vi "raise Height state.vi"(8 "Write Height":dbl, 9 "Write":bool, 11 "Enum":enum16{"read", "write"}(ring)) -> (0 "read Height":dbl, 1 "read":bool)   [LabVIEW 2019]
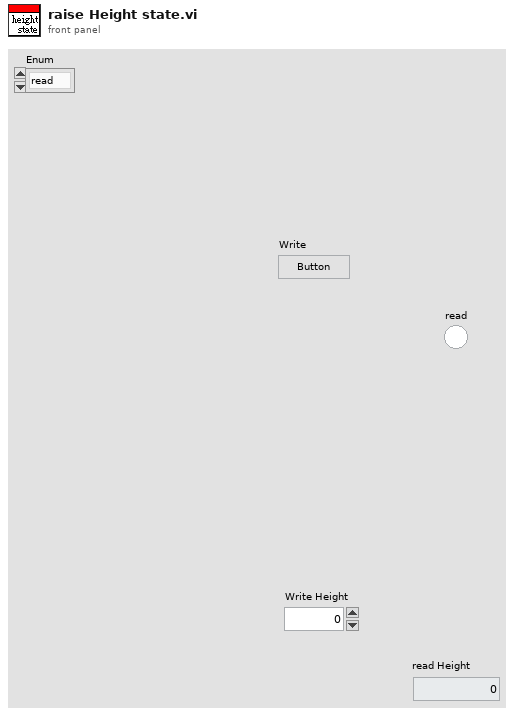
[diagram p1: front panel]
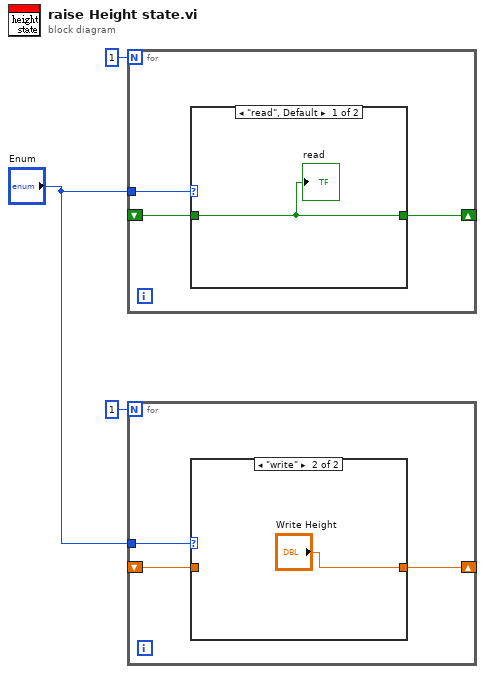
[diagram p0: block diagram]
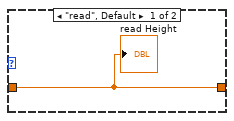
[diagram p2: hidden frame]
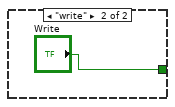
[diagram p3: hidden frame]
diagram:
  n1 = for {
    N: 1 -> [_]
    shift-right: [w5] -> _
    shift-left: _ -> [w4]
    tunnel: "Enum" -> [w6]
    n2 = case shown="\"read\", Default" w6 {
      tunnel: [w7 "Write"] -> w5
      tunnel: w4 -> [w7 _]
      frame "read", Default {
        "read" <- w7
      }
      frame "write" {
      }
    }
  }
  n3 = for {
    N: 1 -> [_]
    shift-right: [w10] -> _
    shift-left: _ -> [w9]
    tunnel: "Enum" -> [w11]
    n4 = case shown="\"write\"" w11 {
      tunnel: [w12 "Write Height"] -> w10
      tunnel: w9 -> [w12 _]
      frame "read", Default {
        "read Height" <- w12
      }
      frame "write" {
      }
    }
  }
